vi "3D-CreateLogFilePath.vi"(11 "路径":path) -> (3 "添加的路径":path)   [LabVIEW 2015]
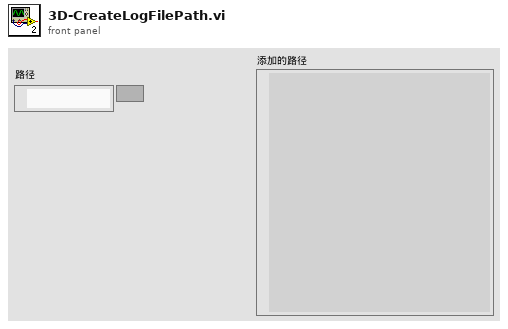
[diagram p1: front panel]
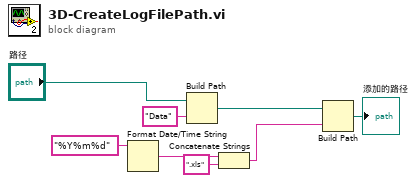
[diagram p0: block diagram]
diagram:
  n1 = Format Date/Time String(time format string (%c)="%Y%m%d" ("时间格式字符串(%c)")) -> (date/time string=w6:string)  [unwired: 2 in]
  n2 = Build Path(base path="路径", name or relative path="Data" ("名称或相对路径")) -> (appended path=w2:path)
  n3 = Concatenate Strings(w6, ".xls" ("字符串")) -> (w4:string)
  n4 = Build Path(base path=w2, name or relative path=w4) -> (appended path=→"添加的路径":path)
